vi "Send Power Meter Detected Message.vi"(0 "Power Meter in":refnum<class "Power Meter Base.lvclass">, 11 "error in":errorcluster) -> (4 "Power Meter out":refnum<class "Power Meter Base.lvclass">, 6 "Active Instrument Info String":string, 15 "error out":errorcluster)   [LabVIEW 2023, in "RFFixtureCharact.Instruments.lvlib" / "Power Meter Factory.lvclass"]
uses:
  Power Meter Factory.lvclass
  Power Meter Base/Power Meter Base.lvclass
  Power Meter Base/Power Meter Base.lvclass/Power Meter Base.ctl
  Power Meter Base/Properties/Read Active Instrument Info.vi
  Common/RFCalAndFixtureCharact.Common.lvlib
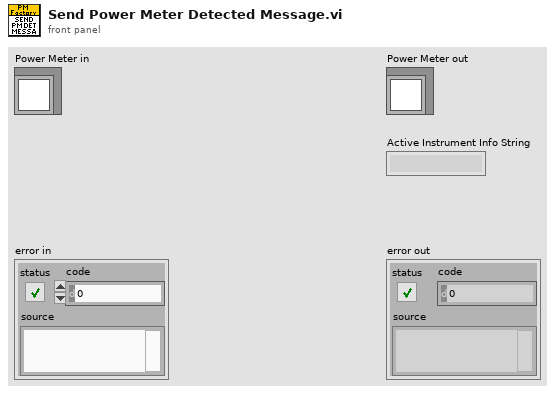
[diagram p1: front panel]
types:
  T1 = typedef "RFFixtureCharact.Instruments.lvlib/Power Meter Base.lvclass/Instrument Info.ctl" = cluster{"User Alias":string, "Resource Name":string, "Product Name":string, "Vendor Name":string}
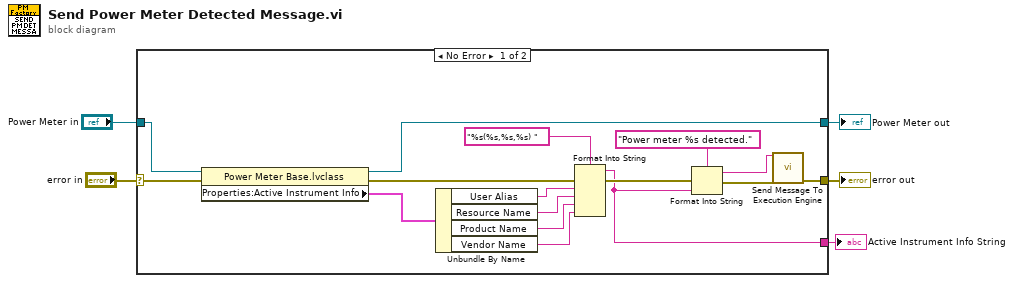
[diagram p0: block diagram]
diagram:
  n1 = case shown="No Error" "error in" {
    selector: "error in" -> [w16 w23]
    tunnel: "Power Meter in" -> [w11 w22]
    tunnel: [w17 w23] -> w5
    tunnel: [w14 w22] -> w3
    tunnel: [w7 _] -> w1
    frame No Error {
      n2 = property class="Power Meter Base.lvclass"(reference=w11, error in=w16) -> (reference out=w14:refnum<class "Power Meter Base.lvclass">, error out=w15:errorcluster, "Properties:Active Instrument Info"=w13:T1)
      n3 = Unbundle By Name(w13) -> ("User Alias"=w18:string, "Resource Name"=w19:string, "Product Name"=w20:string, "Vendor Name"=w21:string)
      n4 = Format Into String(format string="%s(%s,%s,%s) ", error in=w15, w18, w19, w20, w21) -> (resulting string=w7:string, error out=w9:errorcluster)  [unwired: 1 in]
      n5 = Format Into String(format string="Power meter %s detected.", error in=w9, w7) -> (resulting string=w6:string, error out=w8:errorcluster)  [unwired: 1 in]
      n6 = call "Send Message To Execution Engine.vi"("Message"=w6, "error in (no error)"=w8) -> ("error out"=w17:errorcluster)  [unwired: 13 in]
    }
    frame Error {
    }
  }
  "error out" <- w5
  "Power Meter out" <- w3
  "Active Instrument Info String" <- w1
